vi "Read Rack.vi"(8 "error in (no error)":errorcluster, 9 "Point Types":string[](array[string]), 10 "Points":i32[](array[numeric]), 11 "TCP Network Connection in":refnum<k5>) -> (0 "error out":errorcluster, 2 "Array out":sgl[](array[numeric]), 3 "TCP Network Connection out":refnum<k5>)   [LabVIEW 2024, in "OptoMMP.lvlib"]
doc: "Returns an array of analog and digital values read from a single Opto 22 rack. Unoccupied channel values are not displayed.\n\nLast updated: 7/25/2025"
uses:
  <instrlib>/OptoMMP/OptoMMP.lvlib
panel:
  # "Copyright (c) 2025 California Institute of Technology (Caltech).\nU.S. Government sponsorship acknowledged.\n\nLicensed under the Apache License, Version 2.0 (the \"License\");\nyou may not use this file except in compliance with the License.\nYou may obtain a copy of the License at\n\n    http://www.apache.org/licenses/LICENSE-2.0\n\nUnless required by applicable law or agreed to in writing, software\ndistributed under the License is distributed on an \"AS IS\" BASIS,\nWITHOUT WARRANTIES OR CONDITIONS OF ANY KIND, either express or implied.\nSee the License for the specific language governing permissions and\nlimitations under the License."
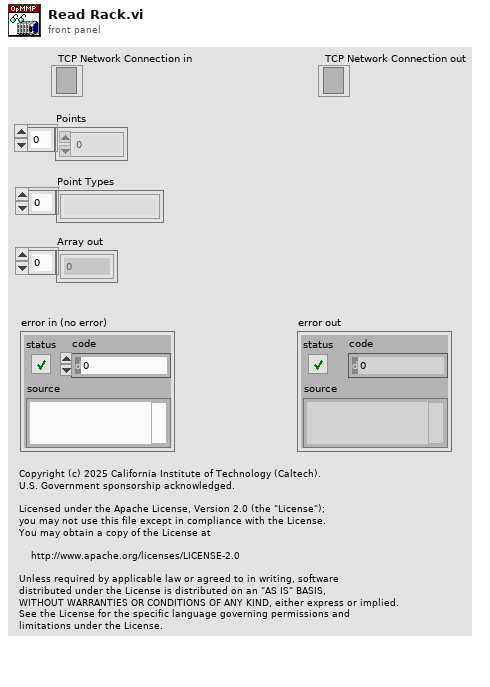
[diagram p1: front panel]
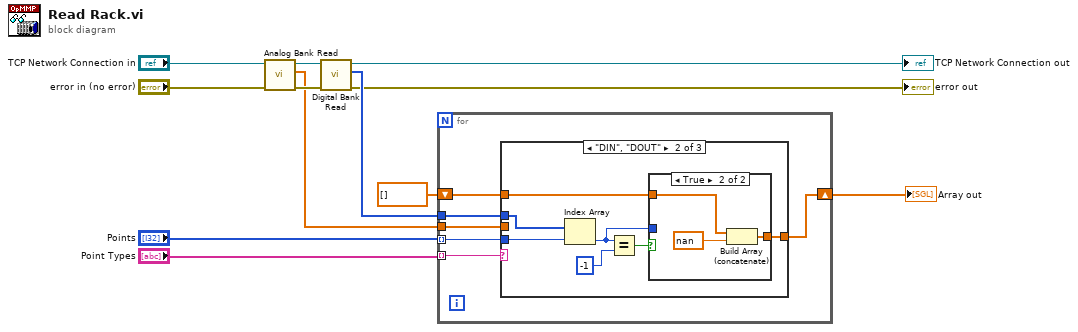
[diagram p0: block diagram]
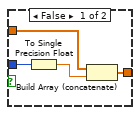
[diagram p3: hidden frame]
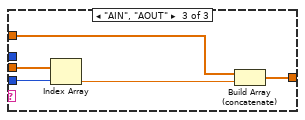
[diagram p4: hidden frame]
diagram:
  n1 = call <instrlib>:"Analog Bank Read.vi"("error in (no error)"="error in (no error)", "TCP Network Connection in"="TCP Network Connection in") -> ("error out"=w9:errorcluster, "Measurements"=w7:sgl[], "TCP Network Connection out"=w8:refnum<k5>)  [unwired: 7 in]
  n2 = call <instrlib>:"Digital Bank Read.vi"("error in (no error)"=w9, "TCP Network Connection in"=w8) -> ("error out"=→"error out":errorcluster, "States"=w10:i16[], "TCP Network Connection out"=→"TCP Network Connection out":refnum<k5>)  [unwired: 7 in]
  n3 = for {
    tunnel: "Point Types" -> [w18] mode=indexing
    tunnel: "Points" -> [w13] mode=indexing
    tunnel: w7 -> [w17]
    tunnel: w10 -> [w16]
    shift-right: [w15] -> w12
    shift-left: sgl[] [] -> [w14]
    n4 = case shown="\"DIN\", \"DOUT\"" w18 {
      tunnel: w17 -> [_ _ w38]
      tunnel: w13 -> [_ w26 w37]
      tunnel: w16 -> [_ w25 _]
      tunnel: [w19 w24 w34] -> w15
      tunnel: w14 -> [w19 w23 w36]
      frame Default {
      }
      frame "DIN", "DOUT" {
        n5 = Index Array(array=w25, index=w26) -> (element=w20:i16)
        n6 = Equal?(x=w20, y=i16 -1) -> (x = y?=w21:bool)
        n7 = case shown="True" w21 {
          tunnel: [w27 w33] -> w24
          tunnel: w23 -> [w28 w32]
          tunnel: w20 -> [w30 _]
          frame False {
            n8 = To Single Precision Float(number=w30) -> (single precision float=w29:sgl)
            n9 = Build Array (concatenate)(w28, w29) -> (w27:sgl[])
          }
          frame True {
            n10 = Build Array (concatenate)(w32, sgl nan) -> (w33:sgl[])
          }
        }
      }
      frame "AIN", "AOUT" {
        n11 = Index Array(array=w38, index=w37) -> (element=w35:sgl)
        n12 = Build Array (concatenate)(w36, w35) -> (w34:sgl[])
      }
    }
  }
  "Array out" <- w12
